vi "Cell I Readback All.vi"(7 "Box ID":u8=1, 8 "error in (no error)":errorcluster, 11 "CAN in":refnum<class "XNET_BS120x.lvclass">) -> (0 "error out":errorcluster, 2 "Current":dbl[](array[numeric]), 3 "CAN out":refnum<class "XNET_BS120x.lvclass">)   [LabVIEW 2021, in "BS120x Driver.lvlib" / "XNET_BS120x.lvclass"]
uses:
  XNET_BS120x.lvclass
  BS120x.lvclass
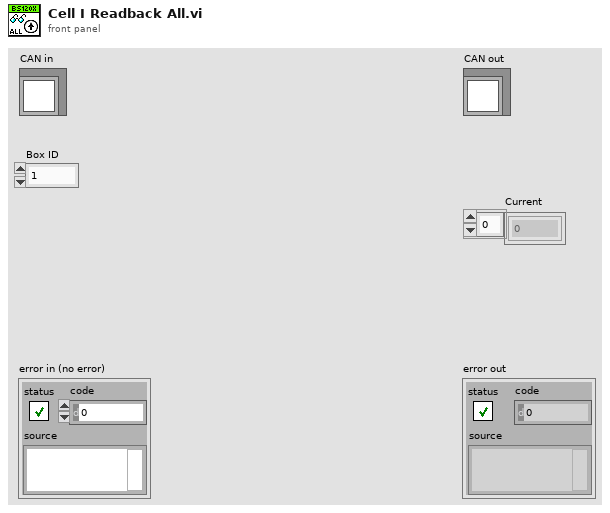
[diagram p1: front panel]
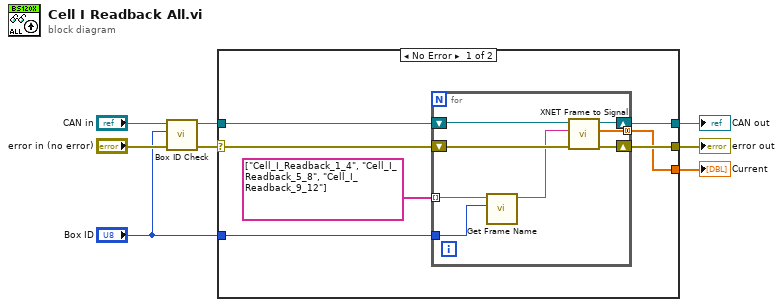
[diagram p0: block diagram]
diagram:
  n1 = call "Box ID Check.vi"("error in (no error)"="error in (no error)", "Box ID"="Box ID", "CAN in"="CAN in") -> ("error out"=w1:errorcluster, "CAN out"=w4:refnum<class "XNET_BS120x.lvclass">)  [unwired: 7 in]
  n2 = case shown="No Error" w1 {
    selector: w1 -> [w9 w25]
    tunnel: w4 -> [w14 w24]
    tunnel: [w13 w24] -> w7
    tunnel: [w12 w25] -> w6
    tunnel: [w11 _] -> w5
    tunnel: "Box ID" -> [w10 _]
    frame No Error {
      n3 = for {
        shift-right: [w20] -> w13
        shift-left: w14 -> [w21]
        shift-right: [w22] -> w12
        shift-left: w9 -> [w23]
        tunnel: [w19] -> w11 mode=concatenating
        tunnel: string[] ["Cell_I_Readback_1_4", "Cell_I_Readback_5_8", "Cell_I_Readback_9_12"] -> [w18] mode=indexing
        tunnel: w10 -> [w16]
        n4 = call "Get Frame Name.vi"("Box ID"=w16, "Frame Name"=w18) -> ("Frame Name out"=w17:string)  [unwired: 9 in]
        n5 = call "XNET Frame to Signal.vi"("error in (no error)"=w23, "Frame"=w17, "CAN in"=w21) -> ("error out"=w22:errorcluster, "signal data"=w19:dbl[], "CAN out"=w20:refnum<class "XNET_BS120x.lvclass">)  [unwired: 6 in]
      }
    }
    frame Error {
    }
  }
  "error out" <- w6
  "CAN out" <- w7
  "Current" <- w5
